vi "data_retrieval_processing_queue.vi"() -> ()   [LabVIEW 2021]
uses:
  aedeaee8-9b7f-3fd9-3008-2ee7f98cdf3f.vi
  a5b8f340-0aaf-3fc0-001e-aaef3e36ac3f.vi
panel:
  out "time spent (ms)":u32
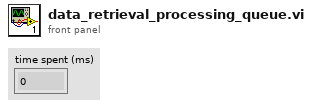
[diagram p1: front panel]
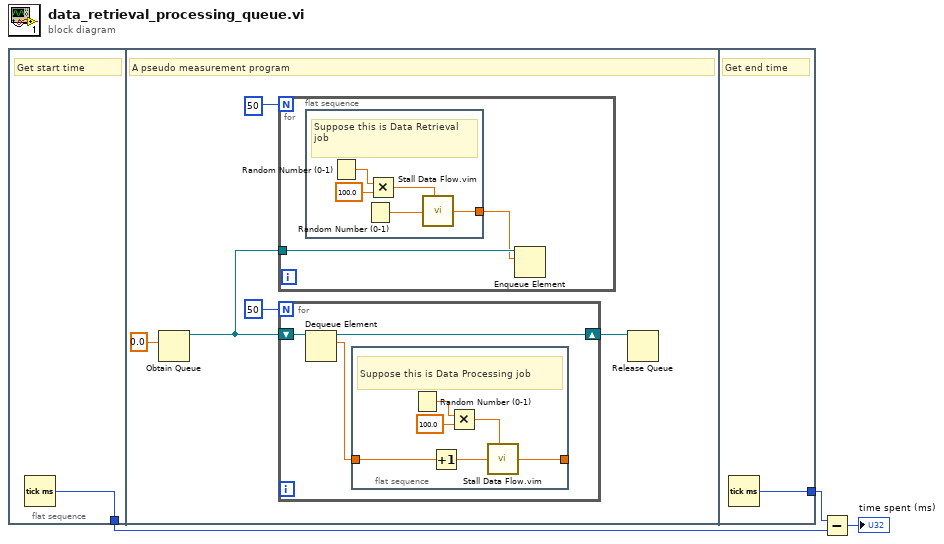
[diagram p0: block diagram]
diagram:
  n1 = flat-sequence {
    tunnel: [w4] -> w2
    tunnel: [w26] -> w3
    frame #0 {
      # "Get start time"
      n2 = Tick Count (ms)() -> (millisecond timer value=w4:u32)
    }
    frame #1 {
      # "A pseudo measurement program"
      n3 = Obtain Queue(element data type=0.0) -> (queue out=w6:refnum<queue>)  [unwired: 4 in, 2 out]
      n4 = for {
        N: 50 -> [_]
        tunnel: w6 -> [w20]
        n5 = flat-sequence {
          tunnel: [w25] -> w19
          frame #0 {
            # "Suppose this is Data Retrieval job"
            n6 = Random Number (0-1)() -> (number: 0 to 1=w24:dbl)
            n7 = Random Number (0-1)() -> (number: 0 to 1=w21:dbl)
            n8 = Multiply(x=w24, y=100.0) -> (x*y=w22:dbl)
            n9 = call "Stall Data Flow.vim"("value in"=w21, "milliseconds to wait"=w22) -> ("value out"=w25:dbl)  [unwired: 1 out]
          }
        }
        n10 = Enqueue Element(queue=w20, element=w19) -> ()  [unwired: 2 in, 3 out]
      }
      n11 = for {
        N: 50 -> [_]
        shift-right: [w10] -> w5
        shift-left: w6 -> [w12]
        n12 = Dequeue Element(queue=w12) -> (queue out=w10:refnum<queue>, element=w11:dbl)  [unwired: 2 in, 2 out]
        n13 = flat-sequence {
          tunnel: [w18] -> _
          tunnel: w11 -> [w13]
          frame #0 {
            # "Suppose this is Data Processing job"
            n14 = Random Number (0-1)() -> (number: 0 to 1=w16:dbl)
            n15 = Increment(x=w13) -> (x+1=w14:dbl)
            n16 = Multiply(x=w16, y=100.0) -> (x*y=w15:dbl)
            n17 = call "Stall Data Flow.vim"("value in"=w14, "milliseconds to wait"=w15) -> ("value out"=w18:dbl)  [unwired: 1 out]
          }
        }
      }
      n18 = Release Queue(queue=w5) -> ()  [unwired: 2 in, 3 out]
    }
    frame #2 {
      # "Get end time"
      n19 = Tick Count (ms)() -> (millisecond timer value=w26:u32)
    }
  }
  n20 = Subtract(x=w3, y=w2) -> (x-y=→"time spent (ms)":u32)
